vi "PROJECTE OCELL versió 0.1.1.vi"() -> ()   [LabVIEW 2020]
uses:
  <vilib>/MakerHub/LINX/LMH-LINX.lvlib
  <vilib>/MakerHub/LINX/Public/Sensors/Distance/Ultrasonic/Ultrasonic.lvlib
  <vilib>/numeric/Random Number (Range) DBL.vi
  <vilib>/MakerHub/LINX/Public/Utilities/Open Serial.vi
  <vilib>/picture/cartesn2.llb/XY Plot Type.ctl
panel:
  out "Distribution Plot":picture
  in  "TEMPS D'ESPERA":i32=30
  in  "JUGADOR 2":dbl
  in  "JUGADOR 1":dbl
  out "appended array":cluster{i32[], dbl[]}[](array[cluster])
  in  "Velocitat de moviment":u32=100
  out "Error Out":errorcluster
  in  "Control d'aturada":bool
  in  "DI Channel":u8
  out "Device Name":string
  in  "Error In":errorcluster
  in  "Baud Rate Override":u32=9600
  in  "Serial Port":refnum<visa-resource-name>="N/A"
  out "Monitor":cluster{i32[], i64[]}[](graph)
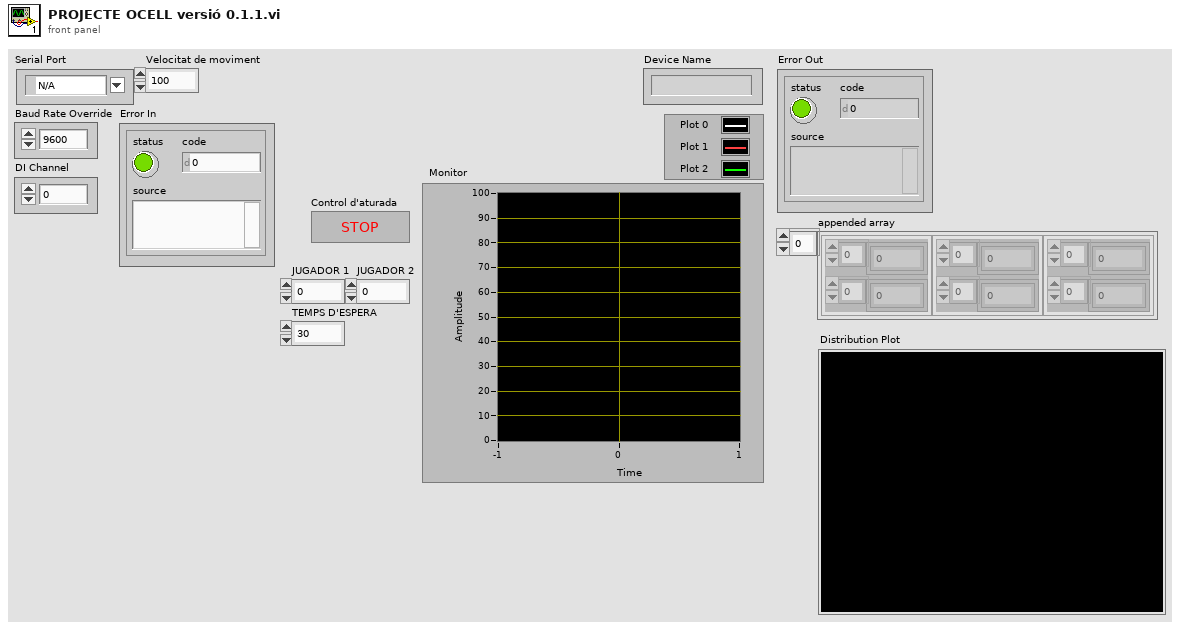
[diagram p1: front panel]
types:
  T1 = cluster{"line color":u32, "text color":u32, "tick length":i16, "crossing axes":bool, "visible grid?":bool}
  T2 = typedef "XY Plot Type.ctl" = enum16{"points", "squares", "circles", "connected points", "connected squares", "connected circles", "comb plot", "sized scatter plot", "sized-colored scatter plot", "min-max lines"}
  T3 = cluster{"plot color":u32, "xy plot type":T2, "baseline":dbl}
  T4 = typedef "LVBoundsTypeDef.ctl" = cluster{"Width":u32, "Height":u32}
  T5 = typedef "LMH-LINX.lvlib/LINX Ref.ctl" = cluster{"IO":T6, "Interface":T7, "LINX Device Config":T8}
  T6 = typedef "LMH-LINX.lvlib/Platform.ctl" = enum16{"Remote", "Local"}
  T7 = typedef "LMH-LINX.lvlib/Interface.ctl" = enum16{"Serial", "TCP"}
  T8 = typedef "LMH-LINX.lvlib/Device.lvlib/LINX Device Config.ctl" = cluster{"Interface":T7, "COM Port":refnum<visa-resource-name>, "TCP Configuration":T9, "Device Family":u8, "Device ID":u8, "Device Name":string, "TCP Ref":refnum<k5>, "Channels":T10}
  T9 = typedef "LMH-LINX.lvlib/Device.lvlib/TCP Config.ctl" = cluster{"IP Address":string, "Port":u16}
  T10 = typedef "LMH-LINX.lvlib/Channels.ctl" = cluster{"DI":u8[], "DO":u8[], "AI":u8[], "AO":u8[], "PWM":u8[], "QE":u8[], "UART":u8[], "I2C 2":u8[], "SPI":u8[], "CAN":u8[], "Servo":u8[], "AI Ref (V)":dbl, "AI Resolution (Bits)":u8, "AO Ref (V)":dbl, "AO Resolution (Bits)":u8}
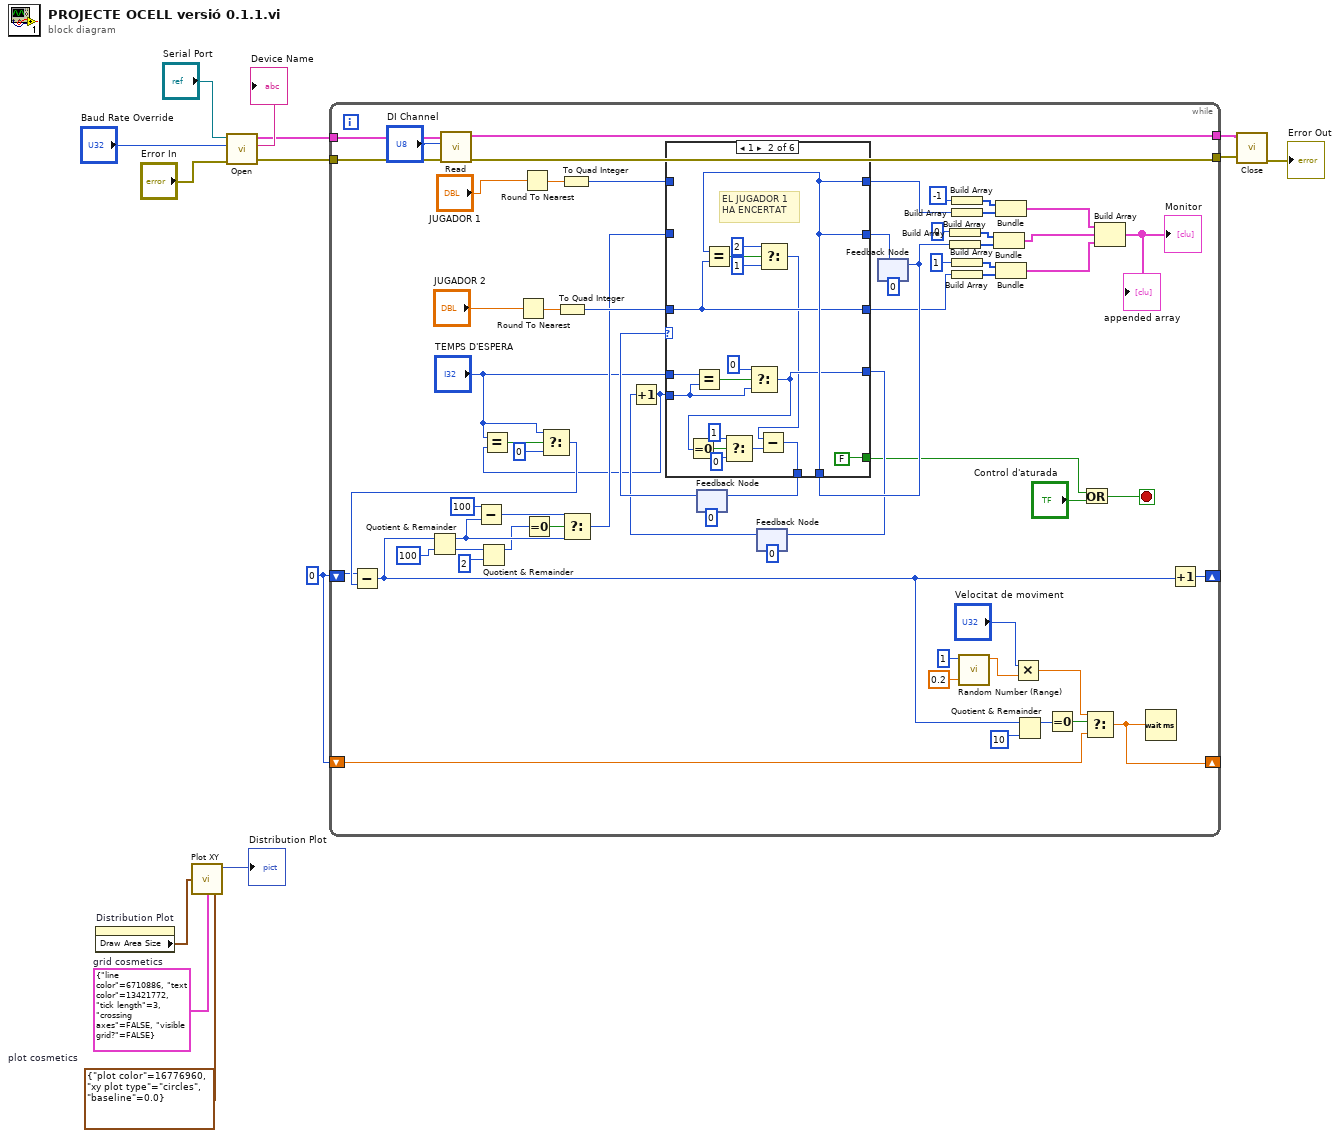
[diagram p0: block diagram]
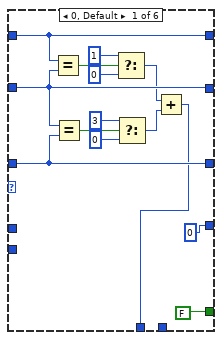
[diagram p2: hidden frame]
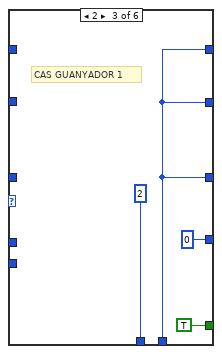
[diagram p3: hidden frame]
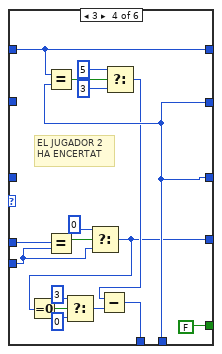
[diagram p4: hidden frame]
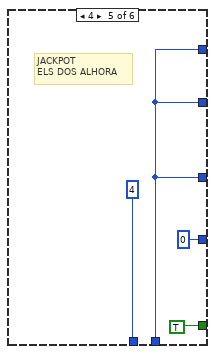
[diagram p5: hidden frame]
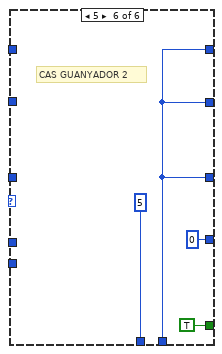
[diagram p6: hidden frame]
diagram:
  w4 = T1 {"line color"=6710886, "text color"=13421772, "tick length"=3, "crossing axes"=FALSE, "visible grid?"=FALSE}  # grid cosmetics
  w3 = T3 {"plot color"=16776960, "xy plot type"=enum."circles", "baseline"=0.0}  # plot cosmetics
  w5 = 0
  n1 = property on="Distribution Plot" class="Pict"() -> ("Draw Area Size"=w2:T4)  [unwired: 2 in, 2 out]
  n2 = call <vilib>:"Plot XY.vi"("dimensions (w,h)"=w2, "cartesian grid cosmetics"=w4, "XY plot cosmetics"=w3) -> ("new picture"=→"Distribution Plot":picture)  [unwired: 12 in]
  n3 = call-poly <vilib>:"Open.vi"("Error In"="Error In", "Baud Rate Override"="Baud Rate Override", "Serial Port"="Serial Port") -> ("Error Out"=w10:errorcluster, "Device Name"=→"Device Name":string, "LINX Resource"=w11:T5)  [unwired: 6 in]
  n4 = while {
    tunnel: w11 -> [w79]
    tunnel: w10 -> [w78]
    tunnel: [w72] -> w9
    tunnel: [w71] -> w8
    shift-right: [w30] -> _
    shift-left: w5 -> [w28]
    shift-right: [w15] -> _
    shift-left: w5 -> [w16]
    stop <- w38 stop-if-true
    n5 = call <vilib>:"Read.vi"("Error In"=w78, "DI Channel"="DI Channel", "LINX Resource"=w79) -> ("Error Out"=w71:errorcluster, "LINX Resource"=w72:T5)  [unwired: 5 in, 2 out]
    n6 = Round To Nearest(number="JUGADOR 2") -> (nearest integer value=w50:dbl)
    n7 = Round To Nearest(number="JUGADOR 1") -> (nearest integer value=w54:dbl)
    n8 = To Quad Integer(1:w50) -> (0:w46:i64)
    n9 = To Quad Integer(1:w54) -> (0:w53:i64)
    n10 = feedback #1(0 ("f")) -> (w43:i32)
    n11 = feedback #2(0 ("t")) -> (w31:i32)
    n12 = Increment(x=w31) -> (x+1=w26:i32)
    n13 = Equal?(x="TEMPS D'ESPERA", y=w26) -> (x = y?=w33:bool)
    n14 = Select(t="TEMPS D'ESPERA", s=w33, f=0) -> (s? t:f=w29:i32)
    n15 = Subtract(x=w28, y=w29) -> (x-y=w24:i32)
    n16 = Quotient & Remainder(x=w24, y=100) -> (x-y*floor(x/y)=w60:i32, floor(x/y)=w57:i32)
    n17 = Subtract(x=100 ("y"), y=w60) -> (x-y=w59:i32)
    n18 = Quotient & Remainder(x=w57, y=2) -> (x-y*floor(x/y)=w55:i32)  [unwired: 1 out]
    n19 = Equal To 0?(x=w55) -> (x = 0?=w56:bool)
    n20 = Select(t=w59, s=w56, f=w60) -> (s? t:f=w35:i32)
    n21 = feedback #3(0) -> (w48:i32)
    n22 = case shown="1" w43 {
      tunnel: w53 -> [w93 _ _ w128 _ _]
      tunnel: [w93 w107 w113 w128 w134 w138] -> w52
      tunnel: w35 -> [w86 _ _ _ _ _]
      tunnel: [w86 w107 w113 w127 w134 w138] -> w49
      tunnel: w48 -> [_ w107 w113 w127 w134 w138]
      tunnel: w46 -> [w85 w106 _ _ _ _]
      tunnel: [w85 w106 w113 w127 w134 w138] -> w45
      tunnel: [w82 w98 2 ("f") w118 4 ("f") 5 ("f")] -> w44
      tunnel: [FALSE FALSE TRUE FALSE TRUE TRUE] -> w34
      tunnel: w26 -> [_ w102 _ w117 _ _]
      tunnel: [0 ("t") w100 0 ("t") w115 0 ("t") 0 ("t")] -> w37
      tunnel: "TEMPS D'ESPERA" -> [_ w101 _ w116 _ _]
      frame 0, Default {
        n23 = Equal?(x=w93, y=w86) -> (x = y?=w92:bool)
        n24 = Equal?(x=w86, y=w85) -> (x = y?=w89:bool)
        n25 = Select(t=1, s=w92, f=0) -> (s? t:f=w83:i32)
        n26 = Select(t=3, s=w89, f=0) -> (s? t:f=w84:i32)
        n27 = Add(x=w83, y=w84) -> (x+y=w82:i32)
      }
      frame 1 {
        # "EL JUGADOR 1\nHA ENCERTAT"
        n28 = Equal?(x=w101, y=w102) -> (x = y?=w104:bool)
        n29 = Equal?(x=w107, y=w106) -> (x = y?=w110:bool)
        n30 = Select(t=0, s=w104, f=w102) -> (s? t:f=w100:i32)
        n31 = Equal To 0?(x=w100) -> (x = 0?=w96:bool)
        n32 = Select(t=1, s=w96, f=0 ("t")) -> (s? t:f=w97:i32)
        n33 = Select(t=2, s=w110, f=1) -> (s? t:f=w99:i32)
        n34 = Subtract(x=w99, y=w97) -> (x-y=w98:i32)
      }
      frame 2 {
        # "CAS GUANYADOR 1"
      }
      frame 3 {
        # "EL JUGADOR 2\nHA ENCERTAT"
        n35 = Equal?(x=w128, y=w127) -> (x = y?=w131:bool)
        n36 = Equal?(x=w116, y=w117) -> (x = y?=w125:bool)
        n37 = Select(t=0, s=w125, f=w117) -> (s? t:f=w115:i32)
        n38 = Equal To 0?(x=w115) -> (x = 0?=w122:bool)
        n39 = Select(t=3, s=w122, f=0 ("t")) -> (s? t:f=w123:i32)
        n40 = Select(t=5, s=w131, f=3) -> (s? t:f=w119:i32)
        n41 = Subtract(x=w119, y=w123) -> (x-y=w118:i32)
      }
      frame 4 {
        # "JACKPOT\nELS DOS ALHORA"
      }
      frame 5 {
        # "CAS GUANYADOR 2"
      }
    }
    n42 = feedback-in #1(w44) -> ()
    n43 = feedback-in #2(w37) -> ()
    n44 = feedback-in #3(w49) -> ()
    n45 = Build Array(0) -> (w66:i32[])
    n46 = Build Array(w48) -> (w51:i32[])
    n47 = Build Array(-1) -> (w68:i32[])
    n48 = Build Array(w52) -> (w69:i64[])
    n49 = Build Array(1) -> (w64:i32[])
    n50 = Build Array(w45) -> (w63:i64[])
    n51 = call-poly <vilib>:"Random Number (Range).vi"("lower bound (0)"=0.2, "upper bound (100)"=u64 1) -> ("number"=w18:dbl)  [unwired: 9 in]
    n52 = Bundle(w66, w51) -> (w75:cluster{i32[], i32[]})  [unwired: 1 in]
    n53 = Bundle(w68, w69) -> (w76:cluster{i32[], i64[]})  [unwired: 1 in]
    n54 = Bundle(w64, w63) -> (w74:cluster{i32[], i64[]})  [unwired: 1 in]
    n55 = Multiply(x="Velocitat de moviment", y=w18) -> (x*y=w17:dbl)
    n56 = Quotient & Remainder(x=w24, y=10 ("f")) -> (x-y*floor(x/y)=w23:i32)  [unwired: 1 out]
    n57 = Equal To 0?(x=w23) -> (x = 0?=w22:bool)
    n58 = Or(x=w34, y="Control d'aturada") -> (x .or. y?=w38:bool)
    n59 = Select(t=w17, s=w22, f=w16) -> (s? t:f=w15:dbl)
    n60 = Build Array(w76, w75, w74) -> (→"Monitor" →"appended array":cluster{i32[], i64[]}[])
    n61 = Wait (ms)(milliseconds to wait=w15) -> ()  [unwired: 1 out]
    n62 = Increment(x=w24) -> (x+1=w30:i32)
  }
  n63 = call <vilib>:"Close.vi"("Error In"=w8, "LINX Resource"=w9) -> ("Error Out"=→"Error Out":errorcluster)  [unwired: 9 in]
